vi "Joystick Acceleration Limiting.vi"(8 "Loop Time (ms)":dbl=10.0 format="%#_13g", 9 "Rise Time (s)":dbl=0.01 format="%#_13g", 11 "Axes":dbl[](array[numeric])) -> (3 "New Axes Values":dbl[](array[numeric]))   [LabVIEW 2016]
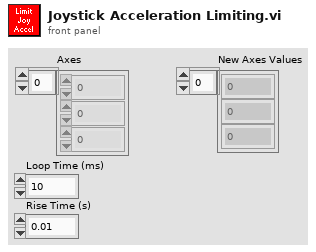
[diagram p1: front panel]
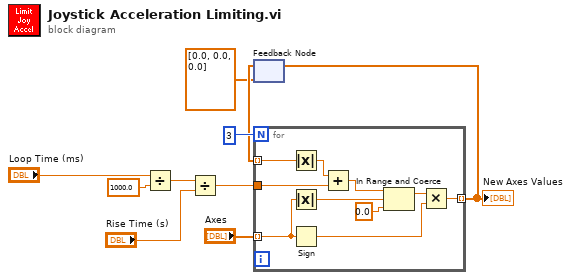
[diagram p0: block diagram]
diagram:
  n1 = Divide(x="Loop Time (ms)", y=1000.0) -> (x/y=w3:dbl)
  n2 = Divide(x=w3, y="Rise Time (s)") -> (x/y=w4:dbl)
  n3 = feedback #1(dbl[] [0.0, 0.0, 0.0]) -> (w8:dbl[])
  n4 = for {
    N: 3 -> [_]
    tunnel: "Axes" -> [w14] mode=indexing
    tunnel: w4 -> [w19]
    tunnel: [w11] -> w7 mode=indexing
    tunnel: w8 -> [w20] mode=indexing
    n5 = Absolute Value(x=w20) -> (abs(x)=w15:dbl)
    n6 = Absolute Value(x=w14) -> (abs(x)=w16:dbl)
    n7 = Sign(1:w14) -> (0:w12:dbl)
    n8 = Add(x=w15, y=w19) -> (x+y=w18:dbl)
    n9 = In Range and Coerce(upper limit=w18, x=w16, lower limit=0.0) -> (coerced(x)=w13:dbl)  [unwired: 1 out]
    n10 = Multiply(x=w13, y=w12) -> (x*y=w11:dbl)
  }
  "New Axes Values" <- w7
  n11 = feedback-in #1(w7) -> ()
